vi "Close.vi"(8 "error in (no error)":errorcluster, 11 "Lamp Container in":refnum<class "Lamp Container.lvclass">) -> (0 "error out":errorcluster, 3 "Lamp Container out":refnum<class "Lamp Container.lvclass">)   [LabVIEW 2016, in "Lamp Container.lvclass"]
uses:
  Lamp Container.lvclass
  Controls/Operational Modes.ctl
  Lamp Container.lvclass/Lamp Container.ctl
  ThAr/ThAr.lvclass
  LED/LED.lvclass
  Quartz/Quartz.lvclass
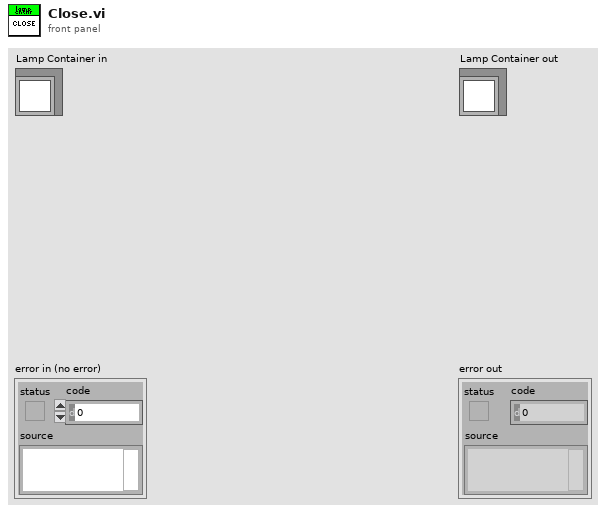
[diagram p1: front panel]
types:
  T1 = typedef "Operational Modes.ctl" = enum16{"Sci", "Sci-LFC", "Solar", "Solar-LFC", "LFC", "LFC-Sim", "LFC-Both", "ThAr", "ThAr-LFC", "Flat", "ExtFlat", "ExtFlat-Sim", "ExtFlat-Both", "Qtz", "ExtQtz", "ExtQtz-Sim", "ExtQtz-Both", "Dark", "Manual", "Off"}
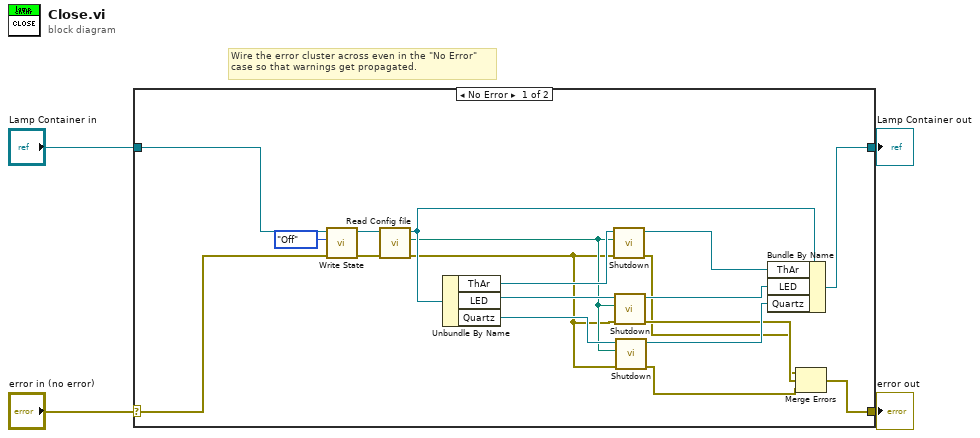
[diagram p0: block diagram]
diagram:
  # "Wire the error cluster across even in the \"No Error\"\ncase so that warnings get propagated."
  n1 = case shown="No Error" "error in (no error)" {
    selector: "error in (no error)" -> [w22 w25]
    tunnel: [w8 w25] -> w3
    tunnel: [w17 w24] -> w1
    tunnel: "Lamp Container in" -> [w23 w24]
    frame No Error {
      n2 = call-dynamic "Write State.vi"("error in (no error)"=w22, "OpMode"=Operational_Modes."Off", "Lamp Container in"=w23) -> ("error out"=w19:errorcluster, "Lamp Container out"=w20:refnum<class "Lamp Container.lvclass">)  [unwired: 7 in]
      n3 = call-dynamic "Read Config file.vi"("error in (no error)"=w19, "Lamp Container in"=w20) -> ("error out"=w11:errorcluster, "Config file"=w12:path, "Lamp Container out"=w18:refnum<class "Lamp Container.lvclass">)  [unwired: 7 in]
      n4 = Unbundle By Name(w18) -> ("ThAr"=w15:refnum<class "ThAr.lvclass">, "LED"=w14:refnum<class "LED.lvclass">, "Quartz"=w13:refnum<class "Quartz.lvclass">)
      n5 = call-dynamic "Shutdown.vi"("error in (no error)"=w11, "config path"=w12, "Lamp in"=w15) -> ("error out"=w5:errorcluster, "Lamp out"=w16:refnum<class "ThAr.lvclass">)  [unwired: 7 in]
      n6 = call-dynamic "Shutdown.vi"("error in (no error)"=w11, "config path"=w12, "Lamp in"=w14) -> ("error out"=w6:errorcluster, "Lamp out"=w10:refnum<class "LED.lvclass">)  [unwired: 7 in]
      n7 = call-dynamic "Shutdown.vi"("error in (no error)"=w11, "config path"=w12, "Lamp in"=w13) -> ("error out"=w7:errorcluster, "Lamp out"=w9:refnum<class "Quartz.lvclass">)  [unwired: 7 in]
      n8 = Bundle By Name(cluster=w18, "ThAr"=w16, "LED"=w10, "Quartz"=w9) -> (w17:refnum<class "Lamp Container.lvclass">)
      n9 = Merge Errors(w5, w6, w7) -> (w8:errorcluster)
    }
    frame Error {
    }
  }
  "error out" <- w3
  "Lamp Container out" <- w1
